vi "ReadMaxAmp.vi"(8 "error in (no error)":errorcluster, 9 "Channel":dbl=1.0, 11 "NI Digitizer in":refnum<class "NI Digitizer.lvclass">) -> (0 "error out":errorcluster, 1 "Amplitude":dbl, 3 "NI Digitizer out":refnum<class "NI Digitizer.lvclass">)   [LabVIEW 2010, in "NI Digitizer.lvclass"]
uses:
  NI Digitizer.lvclass
  <instrlib>/niScope/Controls/niScope scalar measurement.ctl
  NI Digitizer.lvclass/NI Digitizer.ctl
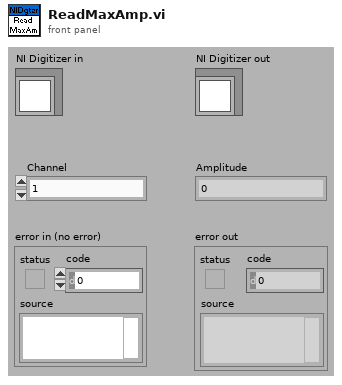
[diagram p1: front panel]
types:
  T1 = typedef "niScope scalar measurement.ctl" = i32
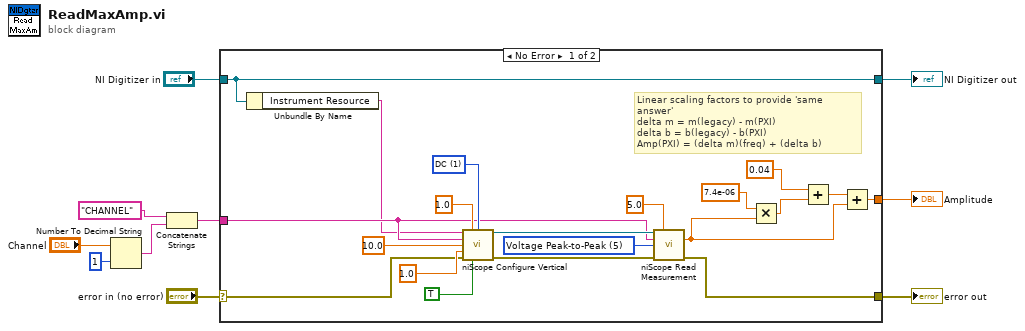
[diagram p0: block diagram]
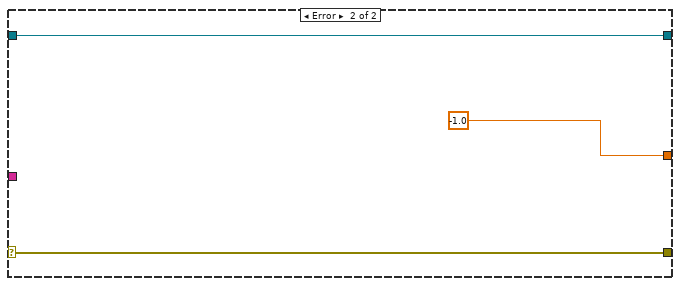
[diagram p2: hidden frame]
diagram:
  n1 = Number To Decimal String(number="Channel", width (-)=i16 1) -> (decimal integer string=w4:string)
  n2 = Concatenate Strings("CHANNEL" ("string"), w4) -> (w2:string)
  n3 = case shown="No Error" "error in (no error)" {
    selector: "error in (no error)" -> [w13 w33]
    tunnel: [w23 w33] -> w9
    tunnel: [w14 -1.0 ("Amplitude")] -> w8
    tunnel: "NI Digitizer in" -> [w12 w31]
    tunnel: [w12 w31] -> w6
    tunnel: w2 -> [w20 _]
    frame No Error {
      w22 = T1 5 items=["None"=4000, "Frequency"=2, "Average Frequency"=1016, "FFT Frequency"=1008, "Period"=3, "Average Period"=1015, "Rise Time"=0, "Fall Time"=1, "Rising Slew Rate"=1010, "Falling Slew Rate"=1011, "Overshoot"=18, "Preshoot"=19, "Voltage RMS"=4, "Voltage Cycle RMS"=16, "AC Estimate"=1012, "FFT Amplitude"=1009, "Voltage Average"=10, "Voltage Cycle Average"=17, "DC Estimate"=1013, "Voltage Max"=6, "Voltage Min"=7, "Voltage Peak-to-Peak"=5, "Voltage High"=8, "Voltage Low"=9, "Voltage Amplitude"=15, "Voltage Top"=1007, "Voltage Base"=1006, "Voltage Base-to-Top"=1017, "Negative Width"=11, "Positive Width"=12, "Negative Duty Cycle"=13, "Positive Duty Cycle"=14, "Integral"=1005, "Area"=1003, "Cycle Area"=1004, "Time Delay"=1014, "Phase Delay"=1018, "Low Ref Volts"=1000, "Mid Ref Volts"=1001, "High Ref Volts"=1002, "Volt. Hist. Mean"=2000, "Volt. Hist. Stdev"=2001, "Volt. Hist. Median"=2003, "Volt. Hist. Mode"=2010, "Volt. Hist. Max"=2005, "Volt. Hist. Min"=2006, "Volt. Hist. Peak-to-Peak"=2002, "Volt. Hist. Mean + Stdev"=2007, "Volt. Hist. Mean + 2 Stdev"=2008, "Volt. Hist. Mean + 3 Stdev"=2009, "Volt. Hist. Hits"=2004, "Volt. Hist. New Hits"=2011, "Time Hist. Mean"=3000, "Time Hist. Stdev"=3001, "Time Hist. Median"=3003, "Time Hist. Mode"=3010, "Time Hist. Max"=3005, "Time Hist. Min"=3006, "Time Hist. Peak-to-Peak"=3002, "Time Hist. Mean + Stdev"=3007, "Time Hist. Mean + 2 Stdev"=3008, "Time Hist. Mean + 3 Stdev"=3009, "Time Hist. Hits"=3004, "Time Hist. New Hits"=3011] ("scalar measurement")
      w28 = 1 items=["AC", "DC", "GND"] ("vertical coupling (DC)")
      # "Linear scaling factors to provide 'same answer'\ndelta m = m(legacy) - m(PXI)\ndelta b = b(legacy) - b(PXI)\nAmp(PXI) = (delta m)(freq) + (delta b)"
      n4 = Unbundle By Name(w12) -> ("Instrument Resource"=w11:string)
      n5 = call <instrlib>:"niScope Configure Vertical.vi"("instrument handle"=w11, "probe attenuation"=1.0, "vertical coupling"=w28, "channels"=w20, "vertical range"=10.0 ("vertical range (10.0 V)"), "vertical offset"=1.0 ("probe attenuation (1:1.0)"), "error in"=w13, "channel enabled"=TRUE) -> ("instrument handle out"=w24:refnum<k15>, "error out"=w25:errorcluster)  [unwired: 1 in, 5 out]
      n6 = call <instrlib>:"niScope Read Measurement.vi"("instrument handle"=w24, "timeout"=5.0, "channels"=w20, "scalar measurement"=w22, "error in"=w25) -> ("result"=w16:dbl, "error out"=w23:errorcluster)  [unwired: 9 out]
      n7 = Multiply(x=7.4e-06 ("element"), y=w16) -> (x*y=w18:dbl)
      n8 = Add(x=0.04 ("element"), y=w18) -> (x+y=w15:dbl)
      n9 = Add(x=w15, y=w16) -> (x+y=w14:dbl)
    }
    frame Error {
    }
  }
  "error out" <- w9
  "NI Digitizer out" <- w6
  "Amplitude" <- w8
